vi "ControlSolenoidShoot.vi"(3 "error in":errorcluster, 4 "task/channels in":refnum<k21>, 5 "On?":bool) -> (0 "error out":errorcluster, 1 "task out":refnum<k21>)   [LabVIEW 2014]
uses:
  <vilib>/DAQmx/write.llb/DAQmx Write (Digital 1D Bool NChan 1Samp 1Line).vi
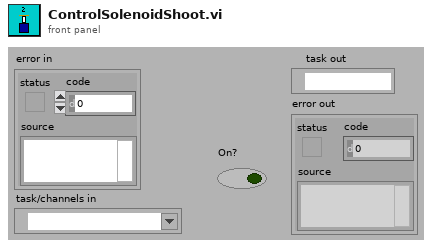
[diagram p1: front panel]
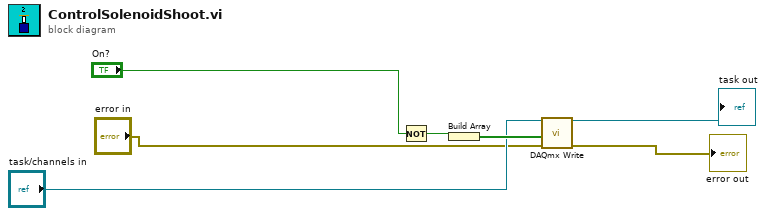
[diagram p0: block diagram]
diagram:
  n1 = Not(x="On?") -> (.not. x?=w6:bool)
  n2 = Build Array(w6) -> (w7:bool[])
  n3 = call-poly <vilib>:"DAQmx Write.vi"("task/channels in"="task/channels in", "data"=w7, "error in"="error in") -> ("task out"=→"task out":refnum<k21>, "error out"=→"error out":errorcluster)  [unwired: 1 in, 10 out]
